vi "自制光源控制.vi"(6 "通道":enum16{"CH1", "CH2", "CH3", "CH4"}(ring), 7 "VISA In":refnum<visa-resource-name>="COM1", 8 "错误输入":errorcluster caption="错误输入（无错误）", 9 "亮度":string="180", 10 "操作模式":enum16{"打开", "关闭", "设置"}(ring), 11 "baud rate":u32=57600) -> (0 "错误输出":errorcluster, 2 "读取缓冲区":string, 3 "VISA Out 2":refnum<visa-resource-name>)   [LabVIEW 2016]
uses:
  <vilib>/Instr/_visa.llb/VISA Configure Serial Port (Instr).vi
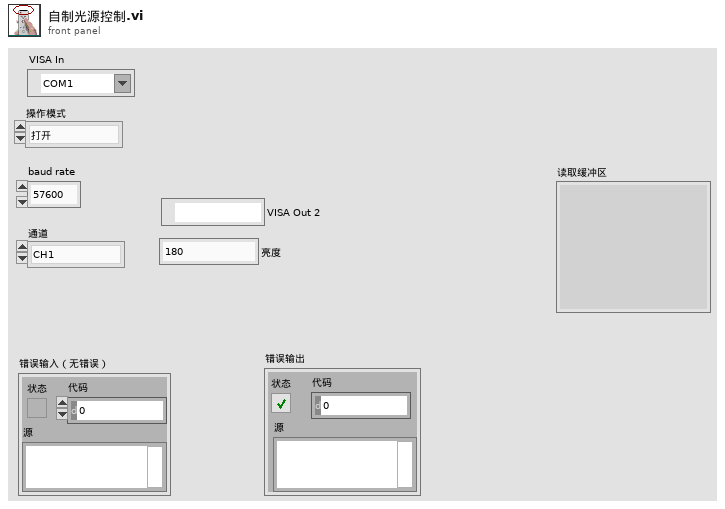
[diagram p1: front panel]
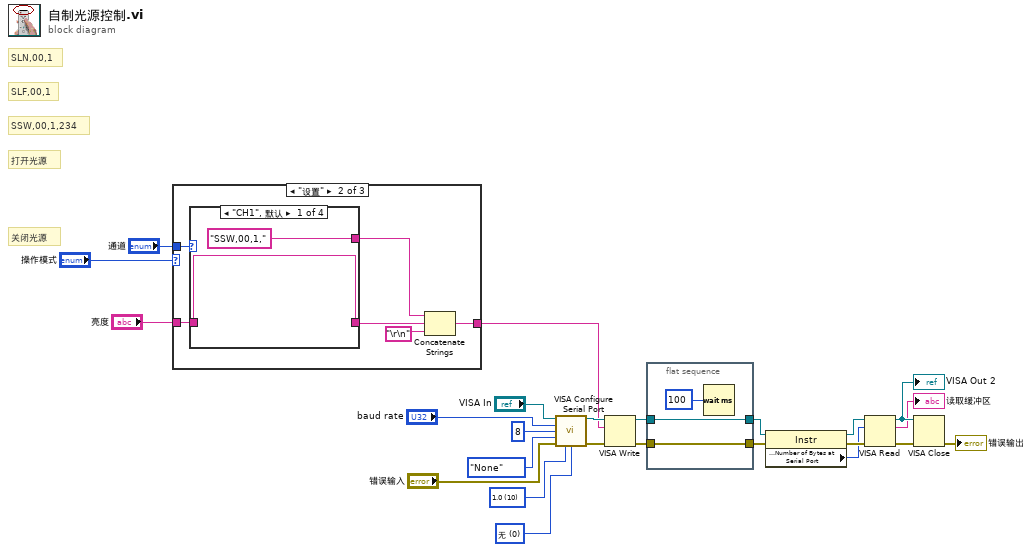
[diagram p0: block diagram]
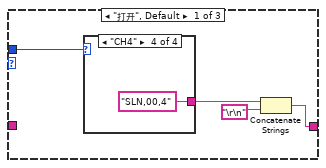
[diagram p2: hidden frame]
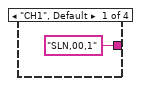
[diagram p3: hidden frame]
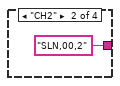
[diagram p4: hidden frame]
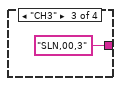
[diagram p5: hidden frame]
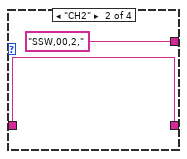
[diagram p6: hidden frame]
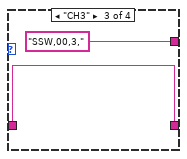
[diagram p7: hidden frame]
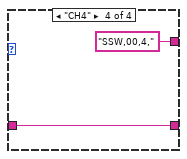
[diagram p8: hidden frame]
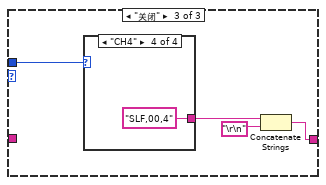
[diagram p9: hidden frame]
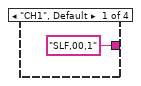
[diagram p10: hidden frame]
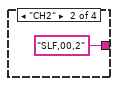
[diagram p11: hidden frame]
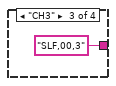
[diagram p12: hidden frame]
diagram:
  w10 = u16 0 items=["无", "XON/XOFF", "RTS/CTS", "XON/XOFF & RTS/CTS", "DTR/DSR", "XON/XOFF & DTR/DSR"] ("flow control (0:none)")
  w11 = u16 10 items=["1.0"=10, "1.5"=15, "2.0"=20] ("stop bits (10: 1 bit)")
  # "SSW,00,1,234"
  # "关闭光源"
  # "打开光源"
  # "SLF,00,1"
  # "SLN,00,1"
  n1 = case shown="\"设置\"" "操作模式" {
    tunnel: [w26 w37 w48] -> w7
    tunnel: "通道" -> [w25 w35 w47]
    tunnel: "亮度" -> [_ w34 _]
    frame "打开", Default {
      n2 = case shown="\"CH4\"" w25 {
        tunnel: ["SLN,00,1" ("写入缓冲区") "SLN,00,2" ("写入缓冲区") "SLN,00,3" ("写入缓冲区") "SLN,00,4" ("写入缓冲区")] -> w28
        frame "CH1", Default {
        }
        frame "CH2" {
        }
        frame "CH3" {
        }
        frame "CH4" {
        }
      }
      n3 = Concatenate Strings(w28, "\r\n" ("行结束常量")) -> (w26:string)
    }
    frame "设置" {
      n4 = case shown="\"CH1\", 默认" w35 {
        tunnel: ["SSW,00,1," ("写入缓冲区") "SSW,00,2," ("写入缓冲区") "SSW,00,3," ("写入缓冲区") "SSW,00,4," ("写入缓冲区")] -> w36
        tunnel: [w39 w41 w43 w45] -> w33
        tunnel: w34 -> [w39 w41 w43 w45]
        frame "CH1", Default {
        }
        frame "CH2" {
        }
        frame "CH3" {
        }
        frame "CH4" {
        }
      }
      n5 = Concatenate Strings(w36, w33, "\r\n" ("行结束常量")) -> (w37:string)
    }
    frame "关闭" {
      n6 = case shown="\"CH4\"" w47 {
        tunnel: ["SLF,00,1" ("写入缓冲区") "SLF,00,2" ("写入缓冲区") "SLF,00,3" ("写入缓冲区") "SLF,00,4" ("写入缓冲区")] -> w50
        frame "CH1", Default {
        }
        frame "CH2" {
        }
        frame "CH3" {
        }
        frame "CH4" {
        }
      }
      n7 = Concatenate Strings(w50, "\r\n" ("行结束常量")) -> (w48:string)
    }
  }
  n8 = call-poly "VISA Configure Serial Port"("VISA resource name"="VISA In", "baud rate (9600)"="baud rate", "data bits (8)"=u16 8, "parity (0:none)"=enum16{"None", "Odd", "Even", "Mark", "Space"}."None", "error in (no error)"="错误输入", "stop bits (10: 1 bit)"=w11, "flow control (0:none)"=w10) -> ("VISA resource name out"=w21:refnum<visa-resource-name>, "error out"=w16:errorcluster)  [unwired: 7 in]
  n9 = VISA Write(VISA resource name=w21, write buffer=w7, error in (no error)=w16) -> (VISA resource name out=w17:refnum<visa-resource-name>, error out=w24:errorcluster)  [unwired: 1 out]
  n10 = flat-sequence {
    tunnel: [w57] -> w22
    tunnel: w17 -> [w57]
    tunnel: [w56] -> w23
    tunnel: w24 -> [w56]
    frame #0 {
      n11 = Wait (ms)(milliseconds to wait=u32 100 ("等待时间（毫秒）")) -> ()  [unwired: 1 out]
    }
  }
  n12 = property class="Instr"(reference=w22, error in=w23) -> (reference out=w5:refnum<visa-resource-name>, error out=w6:errorcluster, "Serial Settings:Number of Bytes at Serial Port"=w4:u32)
  n13 = VISA Read(VISA resource name=w5, byte count=w4, error in (no error)=w6) -> (VISA resource name out=w20:refnum<visa-resource-name>, read buffer=→"读取缓冲区":string, error out=w19:errorcluster)  [unwired: 1 out]
  "VISA Out 2" <- w20
  n14 = VISA Close(VISA resource name=w20, error in (no error)=w19) -> (error out=→"错误输出":errorcluster)
